vi "Fetch Multi Eval Meas List ACLR UTRA Results.vi"(6 "UTRA Channel (First adjacent)":T1=1 items=["First adjacent"=1, "Second adjacent"=2], 7 "Carrier Frequency (Positive)":i32(ring)=1 items=["Negative", "Positive"], 8 "error in (no error)":errorcluster, 9 "Result Type (Current)":i32(ring) items=["Current", "Average"], 10 "Instance (1)":T2=1, 11 "VISA resource name":refnum<visa-resource-name>) -> (0 "error out":errorcluster, 1 "Results":dbl[](array[numeric]) format="%^.3e", 2 "Reliability":i32, 3 "VISA resource name out":refnum<visa-resource-name>)   [LabVIEW 2020, in "Rohde&Schwarz CMWXP NR FR1 Measurement.lvlib"]
doc: "Return the ACLR for the first or second adjacent UTRA channel above (Positive) or below (Negative) the carrier frequency for all measured list mode segments.\n\nAttributes:\nRSCMWXPNRFR1M_ATTR_FETCH_MULTI_EVAL_MEAS_LIST_ACLR_UTRA_NEGATIVE_CURRENT_RESULTS\nRSCMWXPNRFR1M_ATTR_FETCH_MULTI_EVAL_MEAS_LIST_ACLR_UTRA_NEGATIVE_AVERAGE_RESULTS\nRSCMWXPNRFR1M_ATTR_FETCH_MULTI_EVAL_MEAS_LIST_ACLR_UTRA_POSITIVE_CURRENT_RESULTS\nRSCMWXPNRFR1M_ATTR_FETCH_MULTI_EVAL_MEAS_LIST_ACLR_UTRA_POSITIVE_AVERAGE_RESULTS\n\nRemote-control commands:\nFETCh:NRSub:MEAS<i>:MEValuation:LIST:ACLR:UTRA<no>:NEGativ:CURRent?\nFETCh:NRSub:MEAS<i>:MEValuation:LIST:ACLR:UTRA<no>:NEGativ:AVERage?\nFETCh:NRSub:MEAS<i>:MEValuation:LIST:ACLR:UTRA<no>:POSitiv:CURRent?\nFETCh:NRSub:MEAS<i>:MEValuation:LIST:ACLR:UTRA<no>:POSitiv:AVERage?"
uses:
  <instrlib>/Rohde&Schwarz CMWXP NR FR1 Measurement/Rohde&Schwarz CMWXP NR FR1 Measurement.lvlib
  <instrlib>/Rohde&Schwarz CMWXP NR FR1 Measurement/Private/_Instance.ctl
  <instrlib>/Rohde&Schwarz CMWXP NR FR1 Measurement/Private/_UTRA.ctl
  <instrlib>/Rohde&Schwarz CMWXP NR FR1 Measurement/Private/rsidr_core.llb/rsidr_core.lvlib
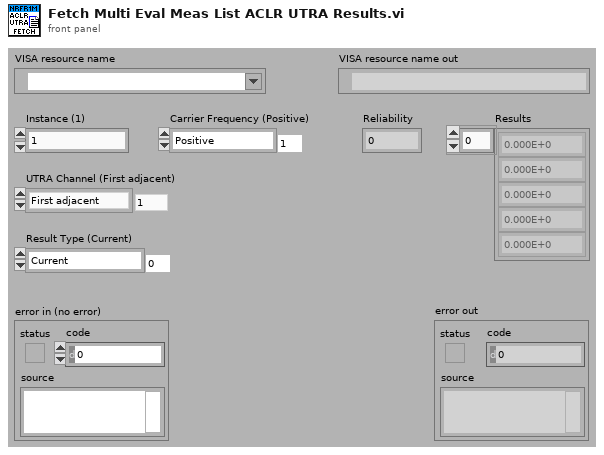
[diagram p1: front panel]
types:
  T1 = typedef "Rohde&Schwarz CMWXP NR FR1 Measurement.lvlib/_UTRA.ctl" = i32
  T2 = typedef "Rohde&Schwarz CMWXP NR FR1 Measurement.lvlib/_Instance.ctl" = i32
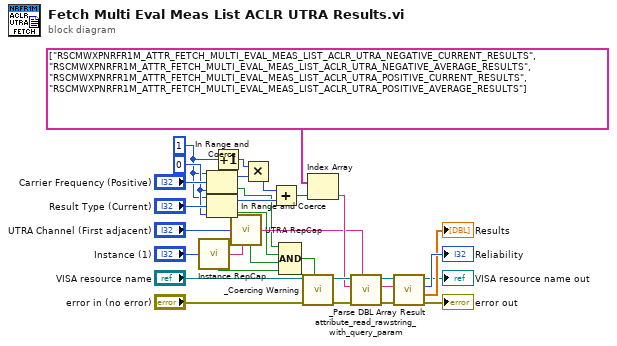
[diagram p0: block diagram]
diagram:
  w5 = 1
  w7 = 0
  n1 = call <instrlib>:"Instance RepCap.vi"("Instance In"="Instance (1)") -> ("In Range?"=w18:bool, "RepCap Identifier Out"=w17:string)  [unwired: 1 in]
  n2 = In Range and Coerce(upper limit=w5, x="Carrier Frequency (Positive)", lower limit=w7) -> (coerced(x)=w6:i32, In Range?=w1:bool)
  n3 = In Range and Coerce(upper limit=w5, x="Result Type (Current)", lower limit=w7) -> (coerced(x)=w9:i32, In Range?=w2:bool)
  n4 = Increment(x=w5) -> (x+1=w4:i32)
  n5 = call <instrlib>:"UTRA RepCap.vi"("UTRA In"="UTRA Channel (First adjacent)", "RepCap String In (\"\")"=w17) -> ("In Range?"=w16:bool, "RepCap Identifier Out"=w15:string)
  n6 = Multiply(x=w4, y=w6) -> (x*y=w3:i32)
  n7 = Add(x=w3, y=w9) -> (x+y=w30:i32)
  n8 = Compound Arithmetic op=AND(w1, w2, w16, w18) -> (w19:bool)
  n9 = call <instrlib>:"_Coercing Warning.vi"("In Range?"=w19, "error in (no error)"="error in (no error)", "VISA resource name"="VISA resource name") -> ("error out"=w27:errorcluster, "VISA resource name out"=w29:refnum<visa-resource-name>)  [unwired: 7 in]
  n10 = Index Array(array=string[] ["RSCMWXPNRFR1M_ATTR_FETCH_MULTI_EVAL_MEAS_LIST_ACLR_UTRA_NEGATIVE_CURRENT_RESULTS", "RSCMWXPNRFR1M_ATTR_FETCH_MULTI_EVAL_MEAS_LIST_ACLR_UTRA_NEGATIVE_AVERAGE_RESULTS", "RSCMWXPNRFR1M_ATTR_FETCH_MULTI_EVAL_MEAS_LIST_ACLR_UTRA_POSITIVE_CURRENT_RESULTS", "RSCMWXPNRFR1M_ATTR_FETCH_MULTI_EVAL_MEAS_LIST_ACLR_UTRA_POSITIVE_AVERAGE_RESULTS"], index=w30) -> (element=w28:string)
  n11 = call <instrlib>:"attribute_read_rawstring_with_query_param.vi"("Repeated Capability"=w15, "error in"=w27, "Attribute ID"=w28, "VISA resource name"=w29) -> ("error out"=w26:errorcluster, "Raw String out"=w25:string, "VISA resource name out"=w24:refnum<visa-resource-name>)  [unwired: 5 in]
  n12 = call <instrlib>:"_Parse DBL Array Result.vi"("error in (no error)"=w26, "Input String"=w25, "VISA resource name"=w24) -> ("error out"=→"error out":errorcluster, "Results"=→"Results":dbl[], "Reliability"=→"Reliability":i32, "VISA resource name out"=→"VISA resource name out":refnum<visa-resource-name>)  [unwired: 5 in]
